vi "Chart.vi"() -> ()   [LabVIEW 2020]
uses:
  AxisReadValues.vi
  SMCD14_lib.lvlib
panel:
  in  "AxisControlSubPanelsArray":refnum<vi>[](array[refnum])
  in  "AxesCount":i32=6
  out "Waveform Chart":T1(graph)
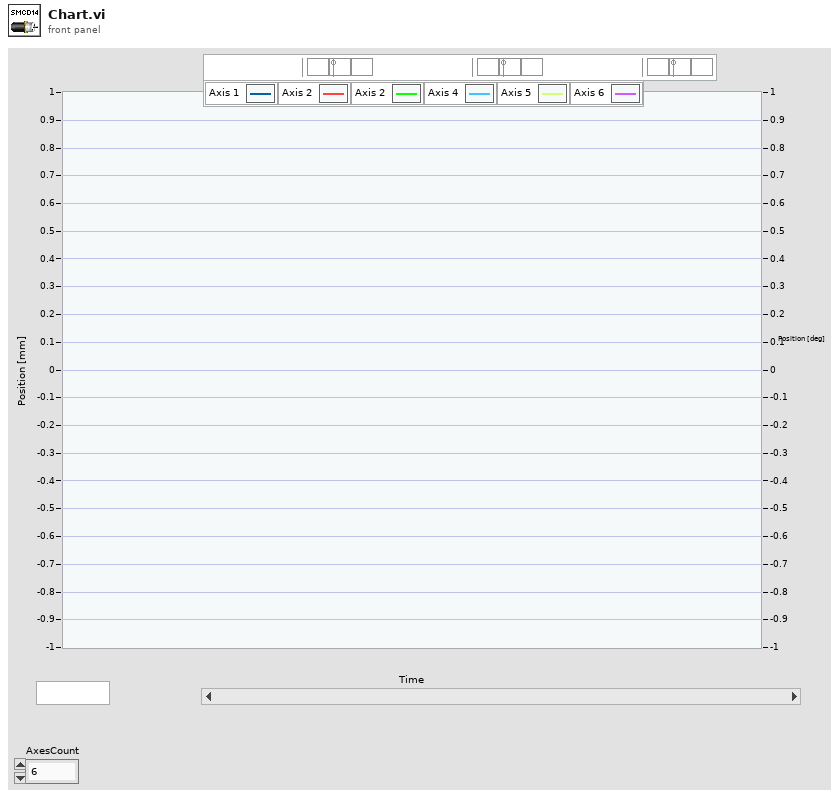
[diagram p1: front panel]
types:
  T1 = cluster{"[0]":dbl, "[1]":dbl, "[2]":dbl, "[3]":dbl, "[4]":dbl, "[5]":dbl, "[6]":dbl, "[7]":dbl, "[8]":dbl}
  T2 = typedef "SMCD14_lib.lvlib/AxisReadValues_typedef.ctl" = cluster{"AxisPosition":dbl, "AxisStatus":i16, "AxisErrorCode":i16, "AxisInPos":bool, "AxisRun":bool, "AxisHomed":bool, "AxisFLS":bool, "AxisBLS":bool, "AxisEnabled":bool, "AxisError":bool, "AxisDog":bool, "AxisVelocity":dbl, "AxisHeartbeat":i16, "SICStatus":i16, "AxisMotorON":bool}
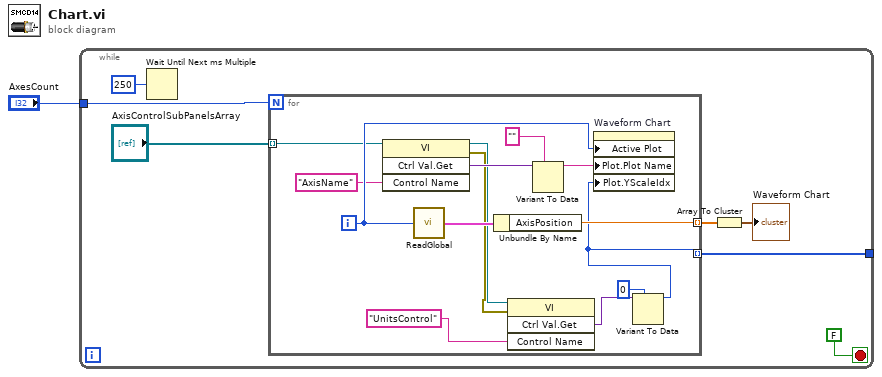
[diagram p0: block diagram]
diagram:
  n1 = while {
    tunnel: "AxesCount" -> [w3]
    tunnel: [w2] -> _
    stop <- FALSE stop-if-true
    n2 = Wait Until Next ms Multiple(millisecond multiple=u32 250) -> ()  [unwired: 1 out]
    n3 = for {
      N: w3 -> [_]
      tunnel: [w21] -> w6 mode=indexing
      tunnel: "AxisControlSubPanelsArray" -> [w19] mode=indexing
      tunnel: [w9] -> w2 mode=indexing
      i -> [w20]
      n4 = invoke class="VI" method="Ctrl Val.Get"(reference=w19, "Control Name"="AxisName") -> (reference out=w14:refnum<vi>, error out=w13:errorcluster, "Get Control Value Variant"=w17:variant)  [unwired: 2 in, 1 out]
      n5 = call-poly "ReadGlobal.vi"("AxisNo"=w20) -> ("AxisReadValuesOUT"=w22:T2)
      n6 = Unbundle By Name(w22) -> ("AxisPosition"=w21:dbl)
      n7 = invoke class="VI" method="Ctrl Val.Get"(reference=w14, error in=w13, "Control Name"="UnitsControl") -> ("Get Control Value Variant"=w10:variant)  [unwired: 1 in, 3 out]
      n8 = Variant To Data(type="" ("Control Name"), Variant=w17) -> (data=w15:string)  [unwired: 1 in, 1 out]
      n9 = Variant To Data(type=0, Variant=w10) -> (data=w9:i32)  [unwired: 1 in, 1 out]
      n10 = property on="Waveform Chart" class="WFChart (strict)"("Active Plot"=w20, "Plot.Plot Name"=w15, "Plot.YScaleIdx"=w9) -> ()  [unwired: 2 in, 2 out]
    }
    n11 = Array To Cluster(array=w6) -> (cluster=→"Waveform Chart":T1)
  }
